vi "TCPIP backup.vi"(0 "SFC":string, 1 "OPERATOR":string, 2 "RESOURCE":string, 3 "NC_CODE":string, 4 "TESTRLT":string, 5 "SERVER":cluster{"IP":string, "PORT":u64, "URL":string}, 6 "SITE":string="X157", 7 "TCP超时":u64=3000, 8 "USER":string="HQ", 9 "error in (no error)":errorcluster caption="错误输入（无错误）", 10 "PWD":string="123456", 11 "抓图？":bool, 12 "STATE":T1(ring)=enum."RLT_PASS", 13 "path to JPEG file":path caption="JPEG文件路径") -> (14 "Y&N":string, 15 "系统消息":string, 19 "error out":errorcluster caption="错误输出")   [LabVIEW 2011]
panel:
  # "http://10.9.30.175:50100\n/manufacturing/IntegrationServlet?InterType=XML&message=\n ERROR<PRODUCTION_REQUEST><NC_LOG_COMPLETE><SITE>A157</SITE><OWNER TYPE=\"USER\">TEST</OWNER><NC_CONTEXT>\n0105442MF01140002</NC_CONTEXT><QTY></QTY><IDENTIFIER></IDENTIFIER><FAILURE_ID></FAILURE_ID><DEFECT_COUNT>1</DEFECT_COUNT>\n<COMMENTS></COMMENTS><DATE_TIME></DATE_TIME><RESOURCE>A-6-Z-TEST</RESOURCE><OPERATION>Z-TEST</OPERATION><ROOT_CAUSE_OPER>\n</ROOT_CAUSE_OPER><NC_CODE>Z-TEST_FAIL</NC_CODE><ACTIVITY>XML</ACTIVITY></NC_LOG_COMPLETE></PRODUCTION_REQUEST>\n!erpautogy03!1234567@byd!ERROR,11V1.0,11V1.0!"
  # "本子VI连接说明如下：\n1)用户验证阶段只需要连接的输入端有USER/PWD/SITE/    SERVER/TCP超时；\n2）条码验证阶段需要连接的输入端有SITE/RESOURCE/OPERATE/USER/   SERVER/TCP超时；\n3）测试结果为PASS,需要连接的输入端有SITE/RESOURCE/OPERATE/USER/SFC/     SERVER/TCP超时；\n4）测试结果为ERROR,.................SITE/RESOURCE/OPERATE/USER/SFC/NC_CODE/    SERVER/TCP超时.\n5)请在STATE枚举中选择所处的阶段。"
  # "[BYD_MES]\nSITE=X157\nOPERATION=Z-CS\nRESOURCE=Z-QT-01-F3-YQ-BLSJQCS-01\nNC_CODE=Z-CS_FAIL\nIP=10.3.3.114\nPORT=50000\nURL=/manufacturing/IntegrationServlet?InterType=XML&message="
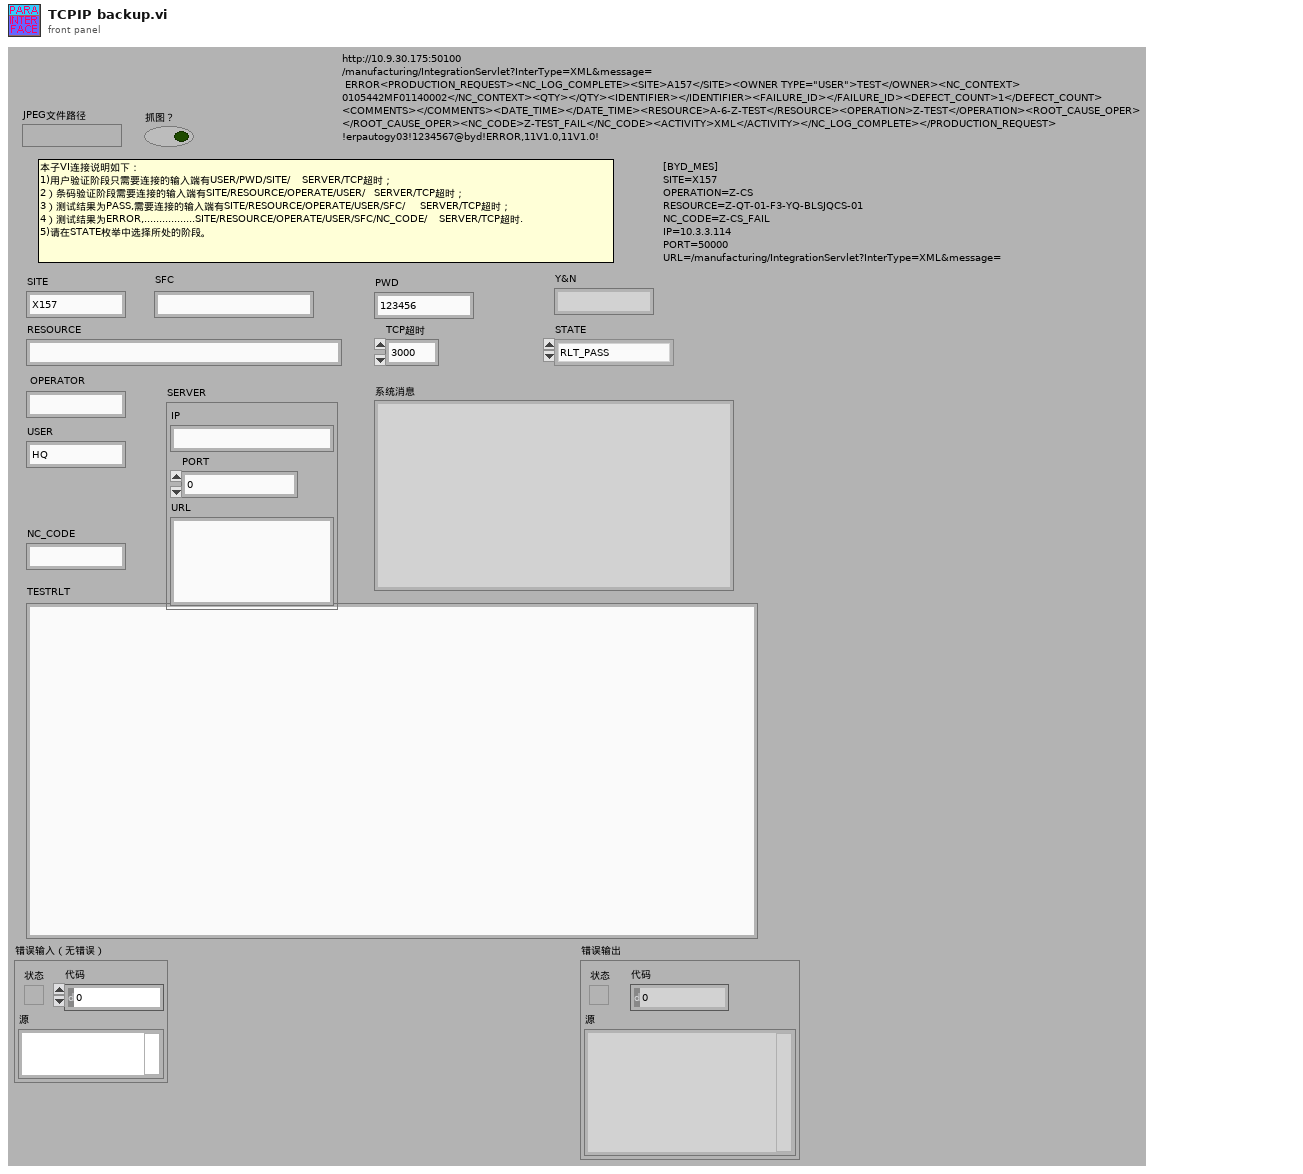
[diagram p1: front panel]
types:
  T1 = enum16{"USER_CHECK", "SFC_CHECK", "RLT_PASS", "RLT_ERROR", "RES_AREA"}
  T2 = cluster{"USER":string, "PWD":string, "SITE":string, "RESOURCE":string, "OPERATOR":string, "NC_CODE":string, "SERVER":cluster{"IP":string, "PORT":u64, "URL":string}}
  T3 = typedef "imagedata.ctl" = cluster{"image type":i32, "image depth":i32, "image":u8[], "mask":u8[], "colors":u32[], "Rectangle":cluster{"left":i16, "top":i16, "right":i16, "bottom":i16}}
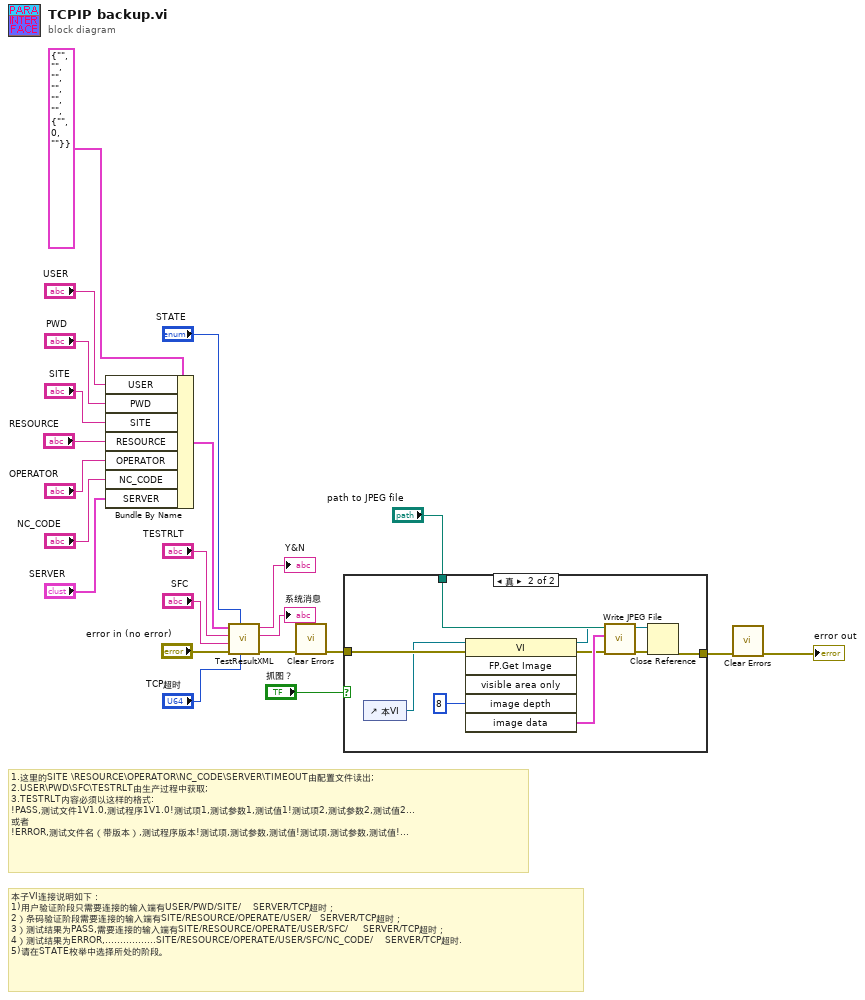
[diagram p0: block diagram]
diagram:
  # "本子VI连接说明如下：\n1)用户验证阶段只需要连接的输入端有USER/PWD/SITE/    SERVER/TCP超时；\n2）条码验证阶段需要连接的输入端有SITE/RESOURCE/OPERATE/USER/   SERVER/TCP超时；\n3）测试结果为PASS,需要连接的输入端有SITE/RESOURCE/OPERATE/USER/SFC/     SERVER/TCP超时；\n4）测试结果为ERROR,.................SITE/RESOURCE/OPERATE/USER/SFC/NC_CODE/    SERVER/TCP超时.\n5)请在STATE枚举中选择所处的阶段。"
  # "1.这里的SITE \\RESOURCE\\OPERATOR\\NC_CODE\\SERVER\\TIMEOUT由配置文件读出;\n2.USER\\PWD\\SFC\\TESTRLT由生产过程中获取;\n3.TESTRLT内容必须以这样的格式:\n!PASS,测试文件1V1.0,测试程序1V1.0!测试项1,测试参数1,测试值1!测试项2,测试参数2,测试值2...\n或者\n!ERROR,测试文件名（带版本）,测试程序版本!测试项,测试参数,测试值!测试项,测试参数,测试值!..."
  n1 = Bundle By Name(cluster=T2 {"USER"="", "PWD"="", "SITE"="", "RESOURCE"="", "OPERATOR"="", "NC_CODE"="", "SERVER"={"IP"="", "PORT"=0, "URL"=""}} ("CONFIG_ITEM"), "USER"="USER", "PWD"="PWD", "SITE"="SITE", "RESOURCE"="RESOURCE", "OPERATOR"="OPERATOR", "NC_CODE"="NC_CODE", "SERVER"="SERVER") -> (w17:T2)
  n2 = call "TestResultXML.vi"("TCP超时"="TCP超时", "STATE"="STATE", "error in (no error)"="error in (no error)", "SFC"="SFC", "TESTRLT"="TESTRLT", "CONFIG_ITEM"=w17) -> ("error out"=w6:errorcluster, "SYSTEM INFO"=→"系统消息":string, "Y&N"=→"Y&N":string)  [unwired: 1 out]
  n3 = call <vilib>:"Clear Errors.vi"("error in (no error)"=w6) -> ("error out"=w1:errorcluster)  [unwired: 6 in]
  n4 = case shown="真" "抓图？" {
    tunnel: w1 -> [w23 w32]
    tunnel: "path to JPEG file" -> [_ w27]
    tunnel: [w23 w24] -> w4
    frame False {
    }
    frame True {
      n5 = control-ref of="本VI"() -> (w31:refnum<vi>)
      n6 = invoke class="VI" method="FP.Get Image"(reference=w31, error in=w32, "image depth"=8 ("图像深度")) -> (reference out=w25:refnum<vi>, error out=w28:errorcluster, "image data"=w29:T3)  [unwired: 3 in, 3 out]
      n7 = call <vilib>:"Write JPEG File.vi"("error in (no error)"=w28, "image data"=w29, "path to JPEG file"=w27) -> ("error out"=w26:errorcluster)  [unwired: 7 in, 1 out]
      n8 = Close Reference(reference=w25, error in (no error)=w26) -> (error out=w24:errorcluster)
    }
  }
  n9 = call <vilib>:"Clear Errors.vi"("error in (no error)"=w4) -> ("error out"=→"error out":errorcluster)  [unwired: 6 in]
